vi "Save_full_Res_rows.vi"(2 "Selected Rows":i32[](array[numeric]), 3 "Filename to write":path, 4 "Filename Orig":path) -> ()   [LabVIEW 2015]
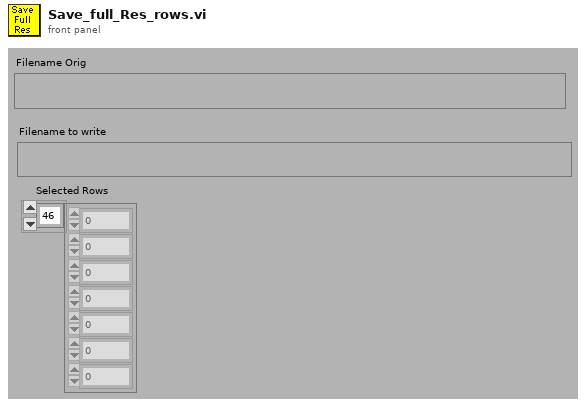
[diagram p1: front panel]
types:
  T1 = enum16{"read/write", "read-only", "write-only", "write-only (truncate)"}
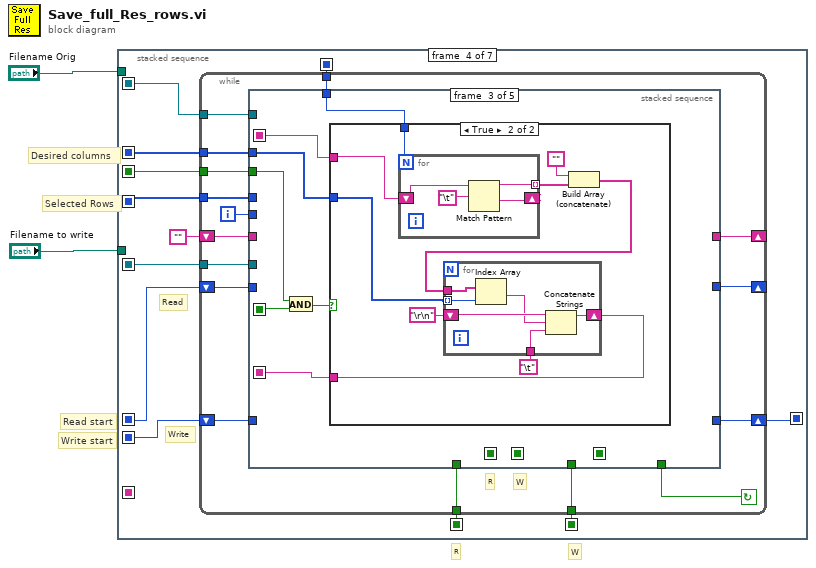
[diagram p0: block diagram]
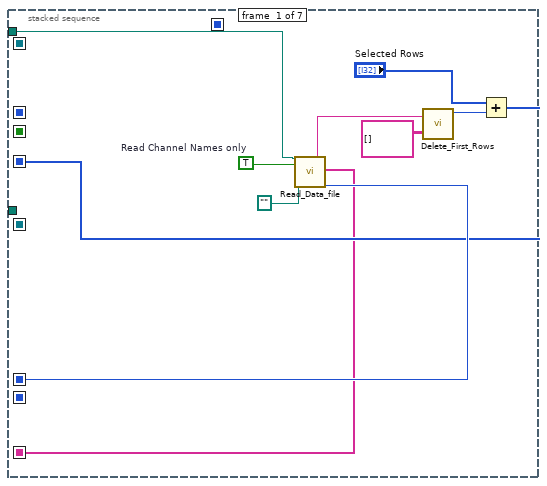
[diagram p2: hidden frame]
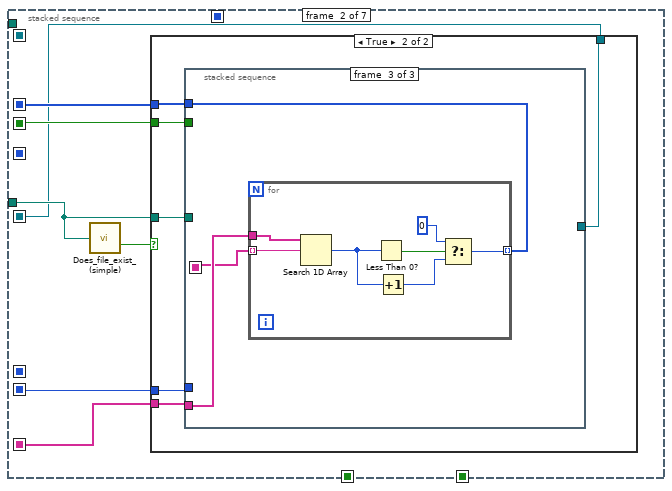
[diagram p3: hidden frame]
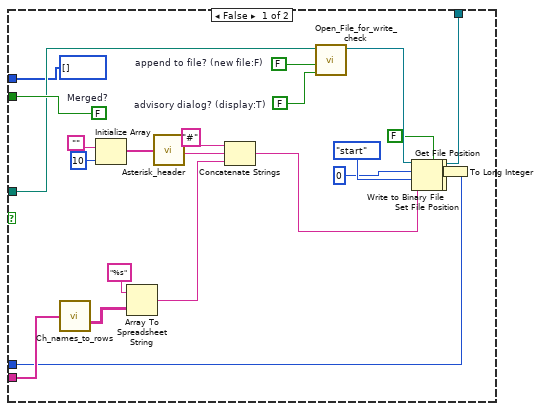
[diagram p4: hidden frame]
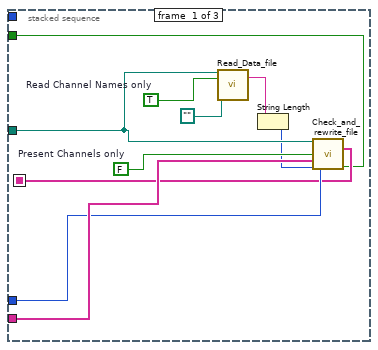
[diagram p5: hidden frame]
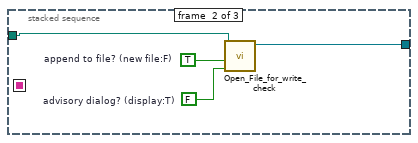
[diagram p6: hidden frame]
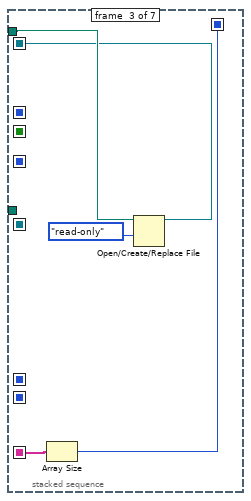
[diagram p7: hidden frame]
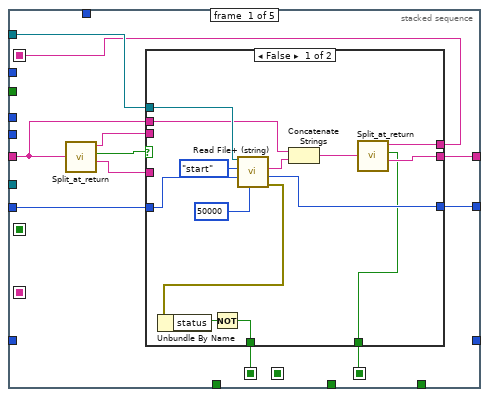
[diagram p8: hidden frame]
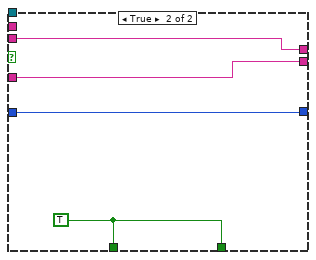
[diagram p9: hidden frame]
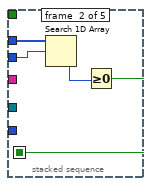
[diagram p10: hidden frame]
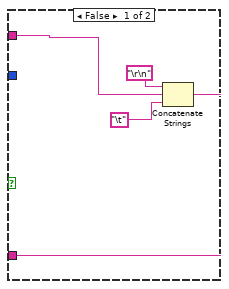
[diagram p11: hidden frame]
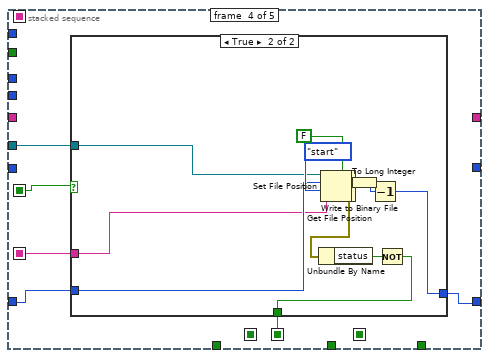
[diagram p12: hidden frame]
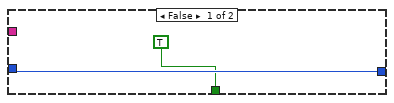
[diagram p13: hidden frame]
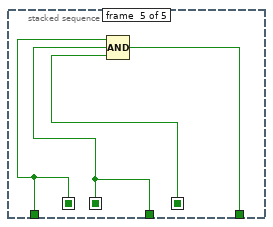
[diagram p14: hidden frame]
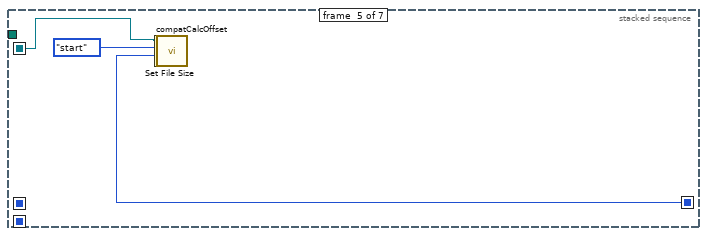
[diagram p15: hidden frame]
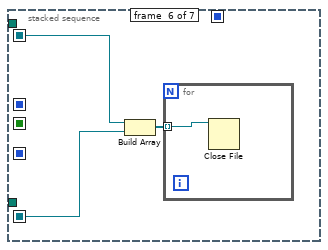
[diagram p16: hidden frame]
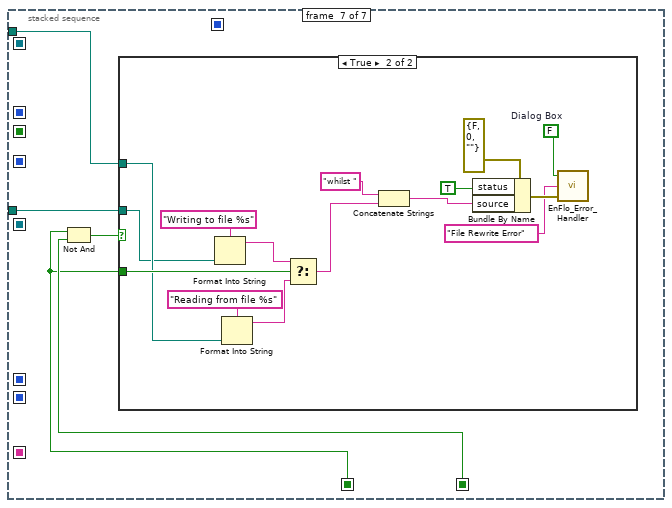
[diagram p17: hidden frame]
diagram:
  # "Desired columns"
  # "Selected Rows"
  # "Read start"
  # "Write start"
  # "W"
  # "R"
  n1 = stacked-sequence {
    seq-local: [_ _ w78 _ _ _ _] -> [_ _ _ w84 _ w207 _]
    seq-local: [w9 _ _ _ _ _ _] -> [_ _ _ w87 _ _ _]
    seq-local: [_ _ _ w91 _ _ _] -> [_ _ _ _ _ _ w211]
    seq-local: [_ _ _ w90 _ _ _] -> [_ _ _ _ _ _ w213]
    seq-local: [_ _ _ w89 _ _ _] -> [_ _ _ _ w204 _ _]
    seq-local: [w4 _ _ _ _ _ _] -> [_ _ _ w88 _ _ _]
    seq-local: [_ w15 _ _ _ _ _] -> [_ _ _ w86 _ _ _]
    seq-local: [w3 _ _ _ _ _ _] -> [_ w18 w77 _ _ _ _]
    seq-local: [_ w17 _ _ _ _ _] -> [_ _ _ w81 _ _ _]
    seq-local: [_ w16 _ _ _ _ _] -> [_ _ _ w82 _ _ _]
    seq-local: [_ w13 _ _ _ _ _] -> [_ _ _ w85 w202 w205 _]
    seq-local: [_ _ w76 _ _ _ _] -> [_ _ _ w83 _ _ _]
    tunnel: "Filename Orig" -> [w10 _ w79 _ _ _ w210]
    tunnel: "Filename to write" -> [_ w14 _ _ _ _ w209]
    frame #0 {
      w11 = TRUE  # Read Channel Names only
      n2 = call "Read_Data_file.vi"("Results file"=w10, "Read Channel Names only"=w11, "Template File"=path "") -> ("Filetype"=w8:string, "Ch names Out"=w3:string[], "mark after read (chars.)"=w9:i32)  [unwired: 2 in, 12 out]
      n3 = call "Delete_First_Rows.vi"("File Type"=w8, "Data In"=string[][] []) -> ("Rows removed"=w7:i32)  [unwired: 2 out]
      n4 = Add(x="Selected Rows", y=w7) -> (x+y=w4:i32[])
    }
    frame #1 {
      n5 = call "Does_file_exist_(simple).vi"("Pathname"=w14) -> ("exists?"=w19:bool)
      n6 = case shown="True" w19 {
        tunnel: w14 -> [w33 w51]
        tunnel: w18 -> [w44 w50]
        tunnel: [i32[] [] w47] -> w17
        tunnel: [w45 w46] -> w16
        tunnel: [w27 w49] -> w15
        tunnel: [w28 w48] -> w13
        frame False {
          w34 = FALSE  # advisory dialog? (display:T)
          w35 = FALSE  # append to file? (new file:F)
          w45 = FALSE  # Merged?
          n7 = call "Ch_names_to_rows.vi"("Channel Names"=w44) -> ("3 Row names"=w37:string[][])
          n8 = Initialize Array("", 10 ("Dimension Size")) -> (w41:string[])
          n9 = Array To Spreadsheet String(array=w37, 3:"%s" ("format string")) -> (spreadsheet string=w36:string)  [unwired: 1 out]
          n10 = call "Asterisk_header.vi"("Channel names"=w41) -> ("Header string"=w40:string)
          n11 = Concatenate Strings("#" ("Substring"), w40, w36) -> (w29:string)
          n12 = call "Open_File_for_write_check.vi"("advisory dialog? (display:T)"=w34, "append to file? (new file:F)"=w35, "file path"=w33) -> ("refnum"=w30:refnum<file>)  [unwired: 8 out]
          n13 = Set File Position(offset (in bytes) (0)=0 ("pos offset (0)"), refnum=w30, from (0:start)=enum16{"start", "end", "current"}."start" ("pos mode (0:2)")) -> (refnum out=w25:refnum<file>, error out=w24:errorcluster)  [unwired: 1 in]
          n14 = Write to Binary File(file (use dialog)=w25, data=w29, error in=w24, 5:FALSE ("prepend array or string size? (T)")) -> (refnum out=w23:refnum<file>, error out=w22:errorcluster)  [unwired: 3 out]
          n15 = Get File Position(4:w22, 7:w23) -> (2:w21:i64, 3:w28:refnum<file>)  [unwired: 1 out]
          n16 = To Long Integer(number=w21) -> (32bit integer=w27:i32)
        }
        frame True {
          n17 = stacked-sequence {
            seq-local: [w58 _ _] -> [_ _ w67]
            tunnel: w51 -> [w54 w63 _]
            tunnel: w50 -> [w60 _ w68]
            tunnel: [w59 _ _] -> w49
            tunnel: [_ w62 _] -> w48
            tunnel: [_ _ w66] -> w47
            tunnel: [w57 _ _] -> w46
            frame #0 {
              w56 = TRUE  # Read Channel Names only
              w61 = FALSE  # Present Channels only
              n18 = call "Read_Data_file.vi"("Results file"=w54, "Read Channel Names only"=w56, "Template File"=path "") -> ("String Before"=w53:string)  [unwired: 2 in, 14 out]
              n19 = String Length(string=w53) -> (length=w52:i32)
              n20 = call "Check_and_rewrite_file.vi"("Filename"=w54, "Present Channels only"=w61, "Present Channels"=w60, "Start of read offset (chars.: 0)"=w52) -> ("Merged Channels"=w58:string[], "Current file size (bytes)"=w59:i32, "Merged?"=w57:bool)  [unwired: 9 out]
            }
            frame #1 {
              w64 = FALSE  # advisory dialog? (display:T)
              w65 = TRUE  # append to file? (new file:F)
              n21 = call "Open_File_for_write_check.vi"("advisory dialog? (display:T)"=w64, "append to file? (new file:F)"=w65, "file path"=w63) -> ("refnum"=w62:refnum<file>)  [unwired: 8 out]
            }
            frame #2 {
              n22 = for {
                tunnel: w68 -> [w75]
                tunnel: w67 -> [w74] mode=indexing
                tunnel: [w69] -> w66 mode=indexing
                n23 = Search 1D Array(1D array=w75, element=w74) -> (index of element=w72:i32)  [unwired: 1 out]
                n24 = Less Than 0?(x=w72) -> (x < 0?=w73:bool)
                n25 = Increment(x=w72) -> (x+1=w71:i32)
                n26 = Select(t=0, s=w73, f=w71) -> (s? t:f=w69:i32)
              }
            }
          }
        }
      }
    }
    frame #2 {
      n27 = Array Size(array=w77) -> (size(s)=w76:i32)
      n28 = Open/Create/Replace File(file path (use dialog)=w79, access (0:read/write)=T1."read-only" ("open mode (0)")) -> (refnum out=w78:refnum<file>)  [unwired: 1 in, 5 out]
    }
    frame #3 {
      # "Write"
      # "Read"
      n29 = while {
        tunnel: [w99] -> w90
        tunnel: [w100] -> w91
        shift-left: w86 -> [w103]
        shift-right: [w102] -> w89
        tunnel: w84 -> [w105]
        shift-left: w87 -> [w107]
        shift-right: [w106] -> _
        shift-left: "" -> [w108]
        shift-right: [w104] -> _
        tunnel: w88 -> [w98]
        tunnel: w85 -> [w96]
        tunnel: w83 -> [w95]
        tunnel: w82 -> [w94]
        tunnel: w81 -> [w93]
        i -> [w97]
        stop <- w101 continue-if-true
        # "R"
        # "W"
        n30 = stacked-sequence {
          seq-local: [w111 _ _ _ _] -> [_ _ w142 _ _]
          seq-local: [_ _ _ w174 _] -> [_ _ _ _ w195]
          seq-local: [w112 _ _ _ _] -> [_ _ _ _ w197]
          seq-local: [w113 _ _ _ _] -> [_ _ _ _ w196]
          seq-local: [_ w138 _ _ _] -> [_ _ w146 w177 _]
          seq-local: [_ _ w147 _ _] -> [_ _ _ w173 _]
          tunnel: w108 -> [w116 _ _ _ _]
          tunnel: w107 -> [w119 _ _ _ _]
          tunnel: [w118 _ _ _ _] -> w106
          tunnel: w105 -> [w117 _ _ _ _]
          tunnel: [w115 _ _ _ _] -> w104
          tunnel: w103 -> [_ _ _ w176 _]
          tunnel: [_ _ _ w175 _] -> w102
          tunnel: [_ _ _ _ w198] -> w101
          tunnel: [_ _ _ _ w196] -> w100
          tunnel: [_ _ _ _ w195] -> w99
          tunnel: w98 -> [_ w141 _ _ _]
          tunnel: w97 -> [_ w140 _ _ _]
          tunnel: w96 -> [_ _ _ w172 _]
          tunnel: w95 -> [_ _ w148 _ _]
          tunnel: w94 -> [_ _ w145 _ _]
          tunnel: w93 -> [_ _ w143 _ _]
          frame #0 {
            n31 = call "Split_at_return.vi"("String"=w116) -> ("before substring"=w110:string, "Matched?"=w109:bool, "after substring"=w114:string)  [unwired: 1 in, 1 out]
            n32 = case shown="False" w109 {
              tunnel: w119 -> [w133 w137]
              tunnel: [w131 w137] -> w118
              tunnel: w117 -> [w130 _]
              tunnel: w116 -> [w128 _]
              tunnel: [w126 w136] -> w115
              tunnel: w114 -> [_ w136]
              tunnel: [w123 w135] -> w113
              tunnel: [w121 w135] -> w112
              tunnel: [w122 w134] -> w111
              tunnel: w110 -> [_ w134]
              frame False {
                n33 = call <vilib>:"Read File+ (string).vi"("count"=50000, "pos offset (bytes:0)"=w133, "pos mode (rel. to current:2)"=enum16{"start", "end", "current"}."start", "refnum"=w130) -> ("error out"=w125:errorcluster, "mark after read (bytes)"=w131:i32, "string"=w129:string)  [unwired: 1 in, 4 out]
                n34 = Unbundle By Name(w125) -> ("status"=w124:bool)
                n35 = Not(x=w124) -> (.not. x?=w123:bool)
                n36 = Concatenate Strings(w128, w129) -> (w127:string)
                n37 = call "Split_at_return.vi"("String"=w127) -> ("before substring"=w122:string, "Matched?"=w121:bool, "after substring"=w126:string)  [unwired: 1 in, 1 out]
              }
              frame True {
                w135 = TRUE
              }
            }
          }
          frame #1 {
            n38 = Search 1D Array(1D array=w141, element=w140) -> (index of element=w139:i32)  [unwired: 1 out]
            n39 = Greater Or Equal To 0?(x=w139) -> (x >= 0?=w138:bool)
          }
          frame #2 {
            n40 = And(x=w145, y=w146) -> (x .and. y?=w144:bool)
            n41 = case shown="True" w144 {
              tunnel: w142 -> [w151 w156]
              tunnel: w143 -> [_ w155]
              tunnel: w148 -> [_ w154]
              tunnel: [w150 w153] -> w147
              frame False {
                n42 = Concatenate Strings("\r\n", w151, "\t") -> (w150:string)
              }
              frame True {
                n43 = for {
                  N: w154 -> [_]
                  shift-right: [w163] -> _
                  shift-left: w156 -> [w164]
                  tunnel: [w162] -> w157 mode=indexing
                  n44 = Match Pattern(string=w164, regular expression="\t") -> (before substring=w162:string, after substring=w163:string)  [unwired: 3 out]
                }
                n45 = Build Array (concatenate)("", w157) -> (w161:string[])
                n46 = for {
                  tunnel: w155 -> [w171] mode=indexing
                  tunnel: w161 -> [w170]
                  shift-right: [w166] -> w153
                  shift-left: "\r\n" -> [w169]
                  tunnel: "\t" -> [w167]
                  n47 = Index Array(array=w170, index=w171) -> (element=w168:string)
                  n48 = Concatenate Strings(w169, w168, w167) -> (w166:string)
                }
              }
            }
          }
          frame #3 {
            n49 = case shown="True" w177 {
              tunnel: w176 -> [w179 w192]
              tunnel: [w179 w191] -> w175
              tunnel: [TRUE w188] -> w174
              tunnel: w173 -> [_ w187]
              tunnel: w172 -> [_ w186]
              frame False {
              }
              frame True {
                n50 = Set File Position(offset (in bytes) (0)=w192, refnum=w186, from (0:start)=enum16{"start", "end", "current"}."start" ("pos mode (0:2)")) -> (refnum out=w185:refnum<file>, error out=w184:errorcluster)  [unwired: 1 in]
                n51 = Write to Binary File(file (use dialog)=w185, data=w187, error in=w184, 5:FALSE ("prepend array or string size? (T)")) -> (refnum out=w183:refnum<file>, error out=w182:errorcluster)  [unwired: 3 out]
                n52 = Get File Position(4:w182, 7:w183) -> (0:w189:errorcluster, 2:w181:i64)  [unwired: 1 out]
                n53 = Unbundle By Name(w189) -> ("status"=w190:bool)
                n54 = To Long Integer(number=w181) -> (32bit integer=w194:i32)
                n55 = Decrement(x=w194) -> (x-1=w191:i32)
                n56 = Not(x=w190) -> (.not. x?=w188:bool)
              }
            }
          }
          frame #4 {
            n57 = Compound Arithmetic op=AND(w196, w195, w197) -> (w198:bool)
          }
        }
      }
    }
    frame #4 {
      n58 = call <vilib>:"compatCalcOffset.vi"("pos offset (0)"=w204, "pos mode (0:1)"=enum16{"start", "end", "current"}."start", "refnum"=w202) -> ("error out"=w201:errorcluster, "offset"=w200:i32, "dup refnum"=w199:refnum<file>)  [unwired: 1 in, 5 out]
      n59 = Set File Size(4:w201, 6:w200, 7:w199) -> ()  [unwired: 2 out]
    }
    frame #5 {
      n60 = Build Array(w207, w205) -> (w206:refnum<file>[])
      n61 = for {
        tunnel: w206 -> [w208] mode=indexing
        n62 = Close File(refnum=w208) -> ()  [unwired: 1 in, 2 out]
      }
    }
    frame #6 {
      n63 = Not And(1:w213, 2:w211) -> (0:w212:bool)
      n64 = case shown="True" w212 {
        tunnel: w211 -> [_ w228]
        tunnel: w210 -> [_ w218]
        tunnel: w209 -> [_ w215]
        frame False {
        }
        frame True {
          w223 = FALSE  # Dialog Box
          n65 = Format Into String(format string="Writing to file %s", w215) -> (resulting string=w214:string)  [unwired: 2 in, 1 out]
          n66 = Format Into String(format string="Reading from file %s", w218) -> (resulting string=w217:string)  [unwired: 2 in, 1 out]
          n67 = Select(t=w214, s=w228, f=w217) -> (s? t:f=w226:string)
          n68 = Concatenate Strings("whilst ", w226) -> (w221:string)
          n69 = Bundle By Name(cluster=errorcluster {"status"=FALSE, "code"=0, "source"=""} ("error in (no error)"), "status"=TRUE ("Bundle Element"), "source"=w221) -> (w224:errorcluster)
          n70 = call "EnFlo_Error_Handler.vi"("error in (no error)"=w224, "Error Type"="File Rewrite Error", "Dialog Box (T)"=w223) -> ()  [unwired: 3 out]
        }
      }
    }
  }
